vi "daq_init.vi"(3 "error in":errorcluster) -> (0 "error out":errorcluster, 1 "Tasks":T1)   [LabVIEW 2011]
uses:
  <vilib>/DAQmx/create/channels.llb/DAQmx Create Channel (AI-Voltage-Basic).vi
  globals.vi
  <vilib>/DAQmx/configure/timing.llb/DAQmx Timing (Sample Clock).vi
  <vilib>/DAQmx/create/channels.llb/DAQmx Create Channel (DO-Digital Output).vi
  <vilib>/DAQmx/create/channels.llb/DAQmx Create Channel (CO-Pulse Generation-Time).vi
  <vilib>/DAQmx/configure/timing.llb/DAQmx Timing (Implicit).vi
  Program Files (x86)/National Instruments/LabVIEW 2011/resource/objmgr/daqmx.rc
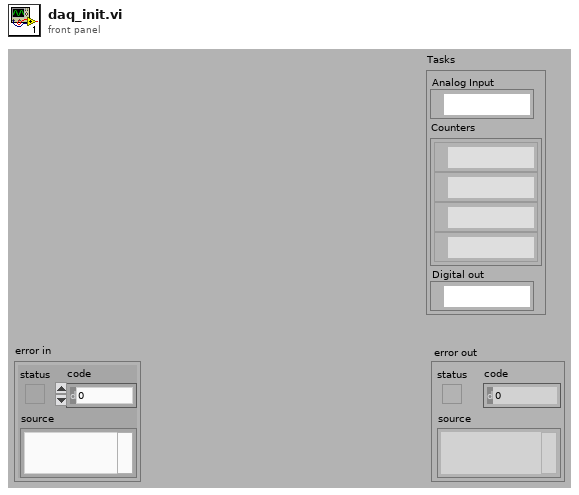
[diagram p1: front panel]
types:
  T1 = cluster{"Analog Input":refnum<k21>, "Counters":refnum<k21>[], "Digital out":refnum<k21>}
  T2 = enum16{"ASAP/Trigger", "ASAP/Finder", "ASAP/Micron", "ASAP/Micron 2", "Micron 6DOF"}
  T3 = cluster{"task out":refnum<k21>, refnum<k21>[], "task out":refnum<k21>}
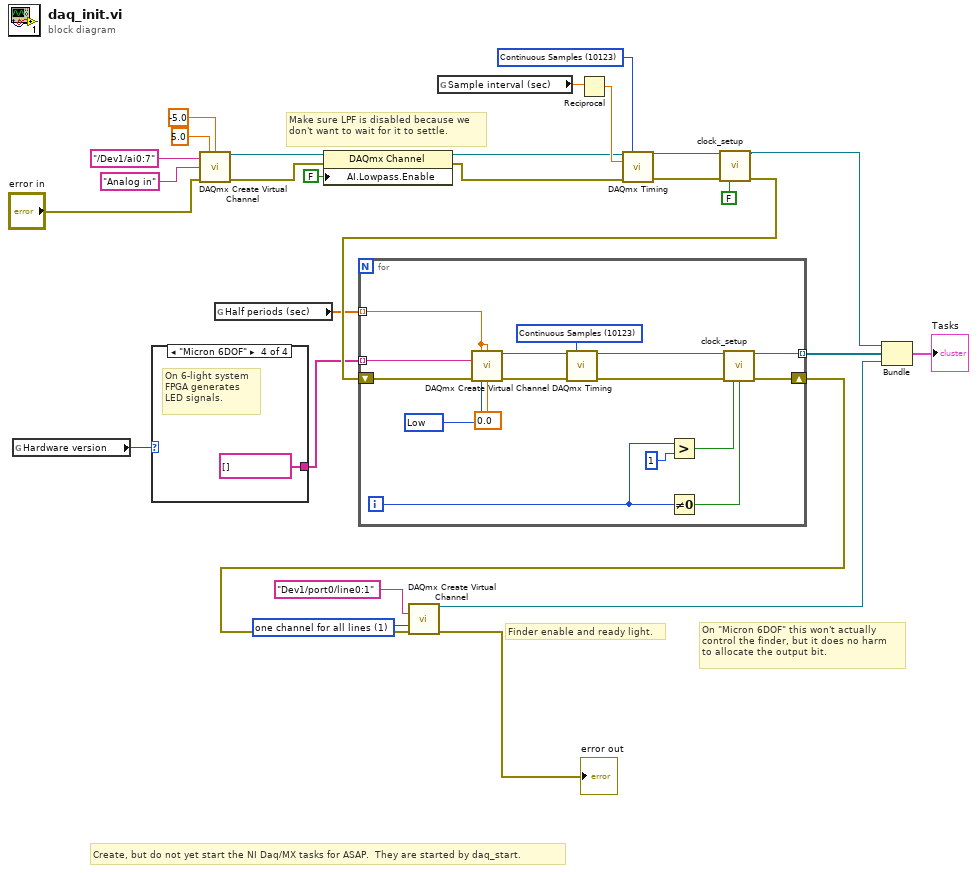
[diagram p0: block diagram]
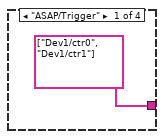
[diagram p2: hidden frame]
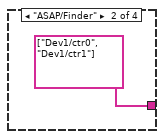
[diagram p3: hidden frame]
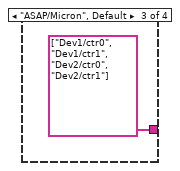
[diagram p4: hidden frame]
diagram:
  w20 = 10123 items=["Finite Samples"=10178, "Continuous Samples"=10123, "Hardware Timed Single Point"=12522] ("sample mode")
  w26 = 1 items=["one channel for each line", "one channel for all lines"] ("line grouping")
  # "Make sure LPF is disabled because we don't want to wait for it to settle."
  # "On \"Micron 6DOF\" this won't actually\ncontrol the finder, but it does no harm\nto allocate the output bit."
  # "Finder enable and ready light."
  # "Create, but do not yet start the NI Daq/MX tasks for ASAP.  They are started by daq_start."
  n1 = global read "globals.vi" "Hardware version"() -> (w11:T2)
  n2 = case shown="\"Micron 6DOF\"" w11 {
    tunnel: [tag[] ["Dev1/ctr0", "Dev1/ctr1"] tag[] ["Dev1/ctr0", "Dev1/ctr1"] tag[] ["Dev1/ctr0", "Dev1/ctr1", "Dev2/ctr0", "Dev2/ctr1"] tag[] []] -> w15
    frame "ASAP/Trigger" {
    }
    frame "ASAP/Finder" {
    }
    frame "ASAP/Micron", Default {
    }
    frame "Micron 6DOF" {
      # "On 6-light system\nFPGA generates \nLED signals."
    }
  }
  n3 = call-poly <vilib>:"DAQmx Create Virtual Channel.vi"("maximum value"=5.0, "minimum value"=-5.0 ("maximum value"), "physical channels"="/Dev1/ai0:7", "name to assign"="Analog in", "error in"="error in") -> ("task out"=w6:refnum<k21>, "error out"=w5:errorcluster)  [unwired: 4 in, 5 out]
  n4 = global read "globals.vi" "Half periods (sec)"() -> (w16:dbl[])
  n5 = property class="DAQmx Channel"(reference=w6, error in=w5, "AI.Lowpass.Enable"=FALSE) -> (reference out=w3:refnum<k21>, error out=w2:errorcluster)
  n6 = global read "globals.vi" "Sample interval (sec)"() -> (w21:dbl)
  n7 = Reciprocal(x=w21) -> (1/x=w19:dbl)
  n8 = call-poly <vilib>:"DAQmx Timing.vi"("task/channels in"=w3, "sample mode"=w20, "rate"=w19, "error in"=w2) -> ("task out"=w9:refnum<k21>, "error out"=w10:errorcluster)  [unwired: 3 in, 7 out]
  n9 = call "clock_setup.vi"("task in"=w9, "error in"=w10, "Dev2"=FALSE) -> ("task out"=w7:refnum<k21>, "error out"=w28:errorcluster)  [unwired: 11 in]
  n10 = for {
    tunnel: w16 -> [w43] mode=indexing
    tunnel: w15 -> [w42] mode=indexing
    shift-right: [w39] -> w14
    shift-left: w28 -> [w41]
    tunnel: [w40] -> w13 mode=indexing
    i -> [w35]
    w46 = 10123 items=["Finite Samples"=10178, "Continuous Samples"=10123] ("sample mode")
    w47 = 10214 items=["High"=10192, "Low"=10214] ("Idle State")
    n11 = call-poly <vilib>:"DAQmx Create Virtual Channel.vi"("high time"=w43, "low time"=w43, "counter"=w42, "error in"=w41, "idle state"=w47, "initial delay"=0.0) -> ("task out"=w45:refnum<k21>, "error out"=w44:errorcluster)  [unwired: 3 in, 5 out]
    n12 = call-poly <vilib>:"DAQmx Timing.vi"("task/channels in"=w45, "sample mode"=w46, "error in"=w44) -> ("task out"=w34:refnum<k21>, "error out"=w33:errorcluster)  [unwired: 1 in, 10 out]
    n13 = Greater?(x=w35, y=1) -> (0:w37:bool)
    n14 = Not Equal To 0?(x=w35) -> (x != 0?=w36:bool)
    n15 = call "clock_setup.vi"("task in"=w34, "error in"=w33, "Dev2"=w37, "Set trigger"=w36) -> ("task out"=w40:refnum<k21>, "error out"=w39:errorcluster)  [unwired: 10 in]
  }
  n16 = call-poly <vilib>:"DAQmx Create Virtual Channel.vi"("lines"="Dev1/port0/line0:1", "line grouping"=w26, "error in"=w14) -> ("task out"=w27:refnum<k21>, "error out"=→"error out":errorcluster)  [unwired: 4 in, 7 out]
  n17 = Bundle("task out"=w7, w13, "task out"=w27) -> (→"Tasks":T3)  [unwired: 1 out]
